vi "Query All Banks.vi"(8 "error in":errorcluster, 11 "ProXR_IO in":refnum<class "ProXR.lvclass">) -> (0 "error out":errorcluster, 2 "Query All Banks":u8[](array[numeric]), 3 "ProXR_IO out":refnum<class "ProXR.lvclass">)   [LabVIEW 2019, in "ProXR.lvlib" / "ProXR.lvclass"]
uses:
  Library/ProXR.lvclass
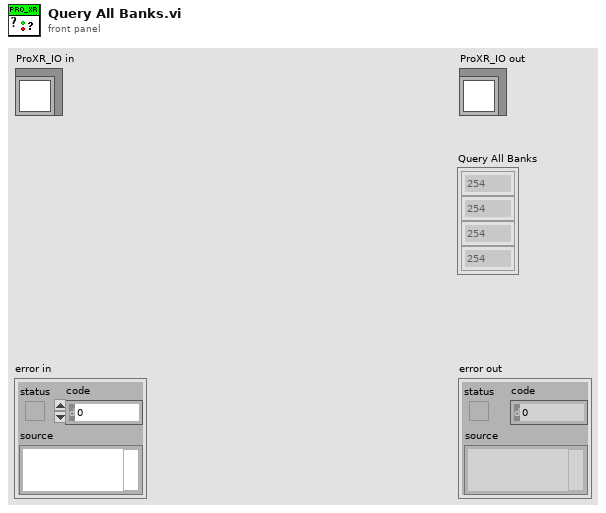
[diagram p1: front panel]
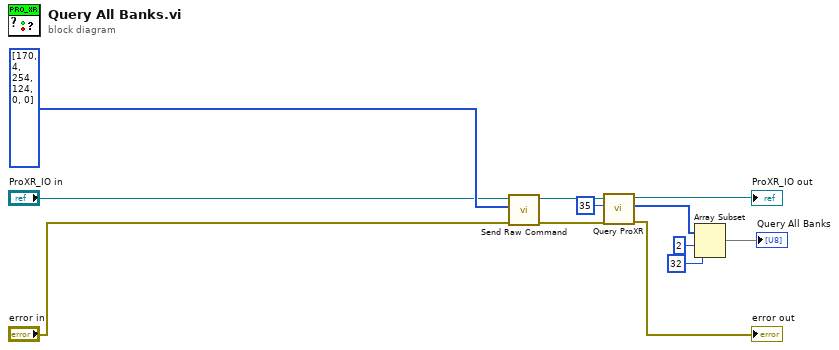
[diagram p0: block diagram]
diagram:
  n1 = call "Send Raw Command.vi"("error in"="error in", "Raw Command"=u8[] [170, 4, 254, 124, 0, 0], "ProXR_IO in"="ProXR_IO in") -> ("error out"=w11:errorcluster, "ProXR_IO out"=w10:refnum<class "ProXR.lvclass">)  [unwired: 7 in]
  n2 = call "Query ProXR.vi"("error in"=w11, "Bytes to Read"=u32 35, "ProXR_IO in"=w10) -> ("error out"=→"error out":errorcluster, "Response"=w5:u8[], "ProXR_IO out"=→"ProXR_IO out":refnum<class "ProXR.lvclass">)  [unwired: 6 in]
  n3 = Array Subset(array=w5, index=2, length=32) -> (→"Query All Banks":u8[])
